vi "close connection.vi"(8 "error in":errorcluster, 11 "ELAN data unit (ADU) in":refnum<class "ELAN Data Unit.lvclass">) -> (0 "error out":errorcluster, 3 "ELAN data unit (ADU) out":refnum<class "ELAN Data Unit.lvclass">)   [LabVIEW 2021, in "ELAN Data Unit.lvclass"]
doc: "This provides an interface for the master to close a connection to the slave."
uses:
  ELAN Data Unit.lvclass
  ELAN Data Unit.lvclass/ELAN Data Unit.ctl
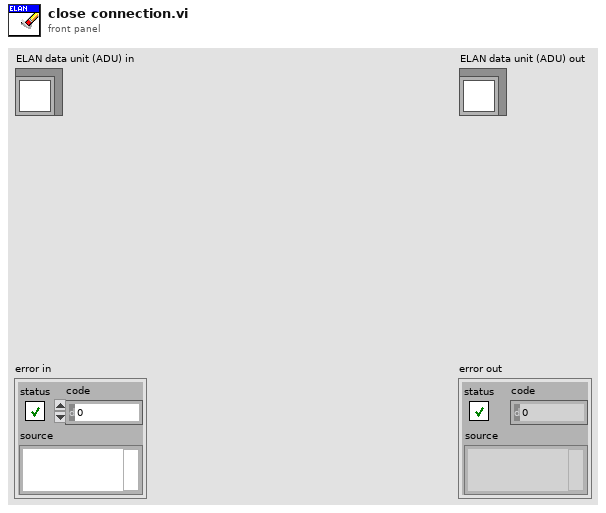
[diagram p1: front panel]
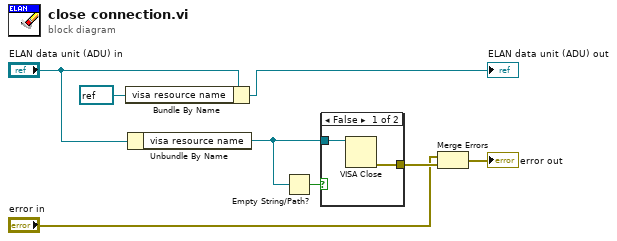
[diagram p0: block diagram]
diagram:
  n1 = Bundle By Name(cluster="ELAN data unit (ADU) in", "visa resource name"=refnum<visa-resource-name> refnum ("VISA resource name")) -> (→"ELAN data unit (ADU) out":refnum<class "ELAN Data Unit.lvclass">)
  n2 = Unbundle By Name("ELAN data unit (ADU) in") -> ("visa resource name"=w3:refnum<visa-resource-name>)
  n3 = Empty String/Path?(string/path=w3) -> (empty?=w8:bool)
  n4 = case shown="False" w8 {
    tunnel: [w10 _] -> w7
    tunnel: w3 -> [w9 _]
    frame False {
      n5 = VISA Close(VISA resource name=w9) -> (error out=w10:errorcluster)  [unwired: 1 in]
    }
    frame True {
    }
  }
  n6 = Merge Errors("error in", w7) -> (→"error out":errorcluster)
